vi "בדיקת זמן מיתוג הממסר 7.vi"(8 "error":errorcluster, 11 "Path for Log":path) -> (0 "error out":errorcluster, 1 "בטוח כן/לא":bool, 2 "בדיקת זמן מיתוג הממסר":dbl)   [LabVIEW 2015]
uses:
  <instrlib>/niDMM/nidmm.llb/niDMM Function.ctl
  <instrlib>/niDMM/nidmm.llb/niDMM Resolution in Digits.ctl
  <vilib>/DAQmx/write.llb/DAQmx Write (Digital Bool 1Line 1Point).vi
  <vilib>/DAQmx/create/channels.llb/DAQmx Create Channel (DO-Digital Output).vi
  <instrlib>/niDMM/nidmm.llb/niDMM Configure Measurement Digits.vi
  <vilib>/DAQmx/miscellaneous.llb/DAQmx Fill In Error Info.vi
panel:
  in  "התחל":bool
  # "Right-Click to\nexplain error"
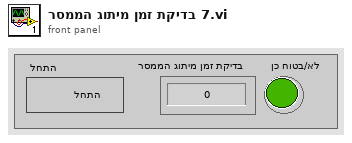
[diagram p1: front panel]
types:
  T1 = enum32{"Invalid", "Standard", "Closed", "Hidden", "Minimized", "Maximized"}
  T2 = typedef "niDMM Function.ctl" = enum16{"DC Volts", "AC Volts", "DC Current", "AC Current", "2-wire Resistance", "4-wire Resistance", "Diode", "Frequency", "Period", "AC Volts DC Coupled", "Capacitance", "Inductance", "Temperature"}
  T3 = typedef "niDMM Resolution in Digits.ctl" = dbl
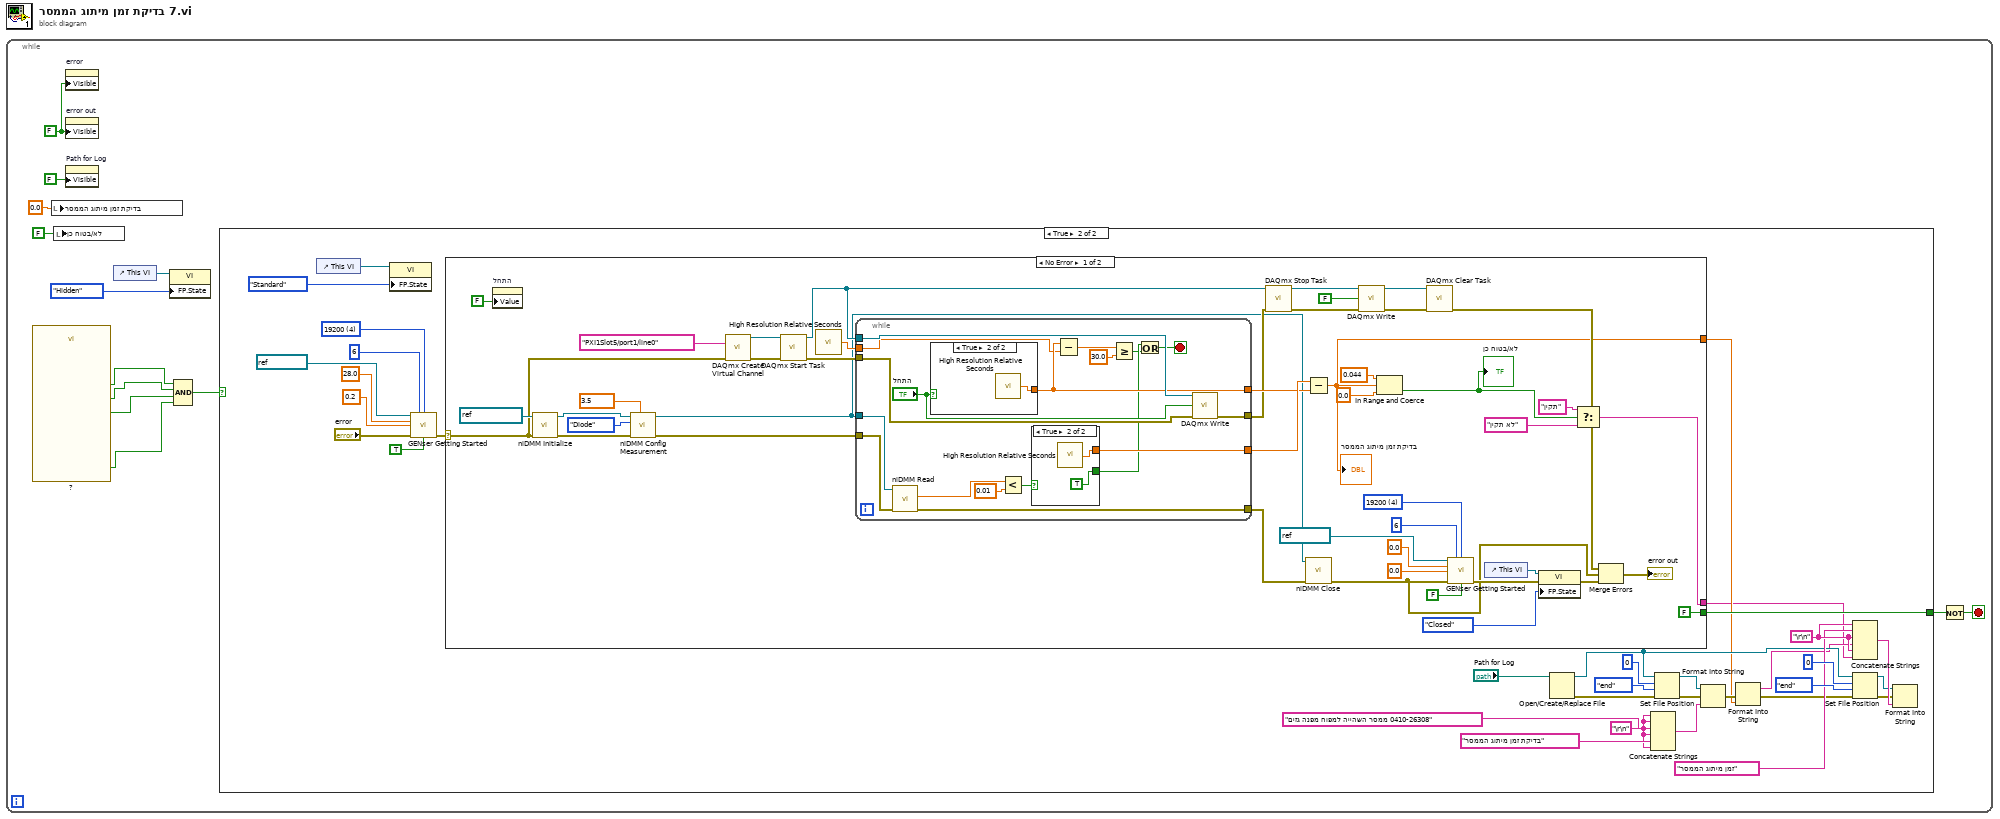
[diagram p0: block diagram]
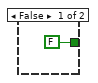
[diagram p2: hidden frame]
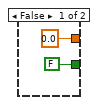
[diagram p3: hidden frame]
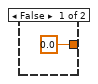
[diagram p4: hidden frame]
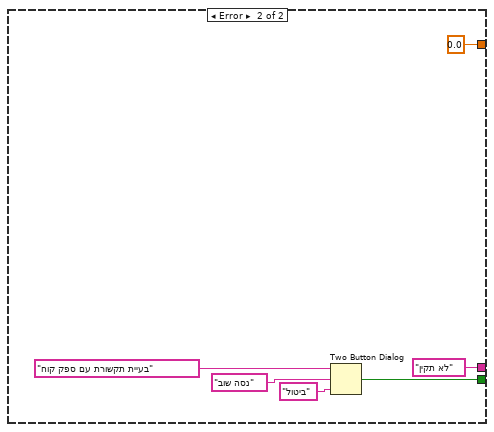
[diagram p5: hidden frame]
diagram:
  n1 = while {
    stop <- w11 stop-if-true
    w12 = FALSE ("Visible")
    n2 = call "?"() -> ("הדקי הרב מודד"=w1:bool, "(מגע שלילי (מעטפת"=w2:bool, "C מגע חיובי"=w3:bool, "OK"=w4:bool)  [unwired: 15 in, 1 out]
    n3 = local write "בדיקת זמן מיתוג הממסר"(0.0 ("בדיקת זמן מיתוג הממסר")) -> ()
    n4 = local write "בטוח כן/לא"(FALSE ("בטוח כן/לא")) -> ()
    n5 = property on="error" class="Clust (strict)"("Visible"=w12) -> ()  [unwired: 2 in, 2 out]
    n6 = property on="error out" class="Clust (strict)"("Visible"=w12) -> ()  [unwired: 2 in, 2 out]
    n7 = property on="Path for Log" class="Path"("Visible"=FALSE) -> ()  [unwired: 2 in, 2 out]
    n8 = control-ref of="This VI"() -> (w10:refnum<vi>)
    n9 = property class="VI"(reference=w10, "FP.State"=T1."Hidden" ("Front Panel Window:State")) -> ()  [unwired: 1 in, 2 out]
    n10 = Compound Arithmetic op=AND(w4, w3, w2, w1) -> (w8:bool)
    n11 = case shown="True" w8 {
      tunnel: [FALSE ("T button?") w41] -> w13
      frame False {
      }
      frame True {
        w25 = "\r\n"
        w32 = "\r\n"
        w44 = u16 4 items=["1200", "2400", "4800", "9600", "19200"] ("BAUD")
        n12 = control-ref of="This VI"() -> (w40:refnum<vi>)
        n13 = property class="VI"(reference=w40, "FP.State"=T1."Standard" ("Front Panel Window:State")) -> ()  [unwired: 1 in, 2 out]
        n14 = call "GENser Getting Started.vi"("VISA"=refnum<visa-resource-name> "COM6", "GEN Addr"=i16 6, "BAUD"=w44, "Voltage Limit"=28.0, "Current Limit"=0.2, "error"="error", "Output On (T)"=TRUE) -> ("error out"=w46:errorcluster)  [unwired: 5 in, 3 out]
        n15 = case shown="No Error" w46 {
          selector: w46 -> [w50 _]
          tunnel: [FALSE ("T button?") w120] -> w41
          tunnel: [w68 0.0] -> w17
          tunnel: [w64 "לא תקין"] -> w16
          frame No Error {
            w56 = T3 3.5 items=["3 1/2"=3.5, "4 1/2"=4.5, "5 1/2"=5.5, "6 1/2"=6.5, "7 1/2"=7.5] ("Resolution in Digits")
            w87 = u16 4 items=["1200", "2400", "4800", "9600", "19200"] ("BAUD")
            n16 = property on="התחל" class="Bool (strict)"("Value"=FALSE ("data")) -> ()  [unwired: 2 in, 2 out]
            n17 = call <instrlib>:"niDMM Initialize.vi"("error in (no error)"=w50, "Instrument Descriptor"=refnum<k15> "PXI1Slot9") -> ("error out"=w54:errorcluster, "instrument handle out"=w55:refnum<k15>)  [unwired: 8 in]
            n18 = call-poly <instrlib>:"niDMM Config Measurement.vi"("Resolution in Digits"=w56, "error in (no error)"=w54, "Function"=niDMM_Function."Diode", "instrument handle"=w55) -> ("error out"=w53:errorcluster, "instrument handle out"=w51:refnum<k15>)  [unwired: 6 in]
            n19 = call-poly <vilib>:"DAQmx Create Virtual Channel.vi"("lines"=tag "PXI1Slot5/port1/line0", "error in"=w50) -> ("task out"=w61:refnum<k21>, "error out"=w62:errorcluster)  [unwired: 12 in]
            n20 = call <vilib>:"DAQmx Start Task.vi"("task/channels in"=w61, "error in"=w62) -> ("task out"=w52:refnum<k21>, "error out"=w59:errorcluster)  [unwired: 12 in]
            n21 = call <vilib>:"High Resolution Relative Seconds.vi"() -> ("relative seconds"=w58:dbl)
            n22 = while {
              tunnel: [w103] -> w76
              tunnel: [w111] -> w77
              tunnel: [w110] -> w75
              tunnel: [w105] -> w74
              tunnel: w52 -> [w109]
              tunnel: w59 -> [w108]
              tunnel: w58 -> [w102]
              tunnel: w53 -> [w95]
              tunnel: w51 -> [w94]
              stop <- w99 stop-if-true
              n23 = call <instrlib>:"niDMM Read.vi"("error in (no error)"=w95, "instrument handle"=w94) -> ("error out"=w105:errorcluster, "Measurement"=w107:dbl)  [unwired: 7 in, 1 out]
              n24 = case shown="True" "התחל" {
                tunnel: [0.0 ("relative seconds") w117] -> w103
                frame False {
                }
                frame True {
                  n25 = call <vilib>:"High Resolution Relative Seconds.vi"() -> ("relative seconds"=w117:dbl)
                }
              }
              n26 = Less?(x=w107, y=0.01) -> (x < y?=w96:bool)
              n27 = case shown="True" w96 {
                tunnel: [0.0 ("relative seconds") w115] -> w111
                tunnel: [FALSE TRUE] -> w98
                frame False {
                }
                frame True {
                  n28 = call <vilib>:"High Resolution Relative Seconds.vi"() -> ("relative seconds"=w115:dbl)
                }
              }
              n29 = Subtract(x=w103, y=w102) -> (x-y=w101:dbl)
              n30 = Greater Or Equal?(x=w101, y=30.0) -> (x >= y?=w97:bool)
              n31 = Or(x=w98, y=w97) -> (x .or. y?=w99:bool)
              n32 = call-poly <vilib>:"DAQmx Write.vi"("task/channels in"=w109, "data"="התחל", "error in"=w108) -> ("error out"=w110:errorcluster)  [unwired: 10 in, 2 out]
            }
            n33 = call <vilib>:"DAQmx Stop Task.vi"("task/channels in"=w52, "error in"=w75) -> ("task out"=w82:refnum<k21>, "error out"=w81:errorcluster)  [unwired: 12 in]
            n34 = Subtract(x=w77, y=w76) -> (x-y=w68:dbl)
            "בדיקת זמן מיתוג הממסר" <- w68
            n35 = call <instrlib>:"niDMM Close.vi"("error in (no error)"=w74, "instrument handle"=w51) -> ("error out"=w49:errorcluster)  [unwired: 9 in]
            n36 = call-poly <vilib>:"DAQmx Write.vi"("task/channels in"=w82, "data"=FALSE, "error in"=w81) -> ("task out"=w79:refnum<k21>, "error out"=w80:errorcluster)  [unwired: 10 in, 1 out]
            n37 = In Range and Coerce(upper limit=0.044, x=w68, lower limit=0.0) -> (In Range?=w65:bool)  [unwired: 1 out]
            "בטוח כן/לא" <- w65
            n38 = call <vilib>:"DAQmx Clear Task.vi"("task in"=w79, "error in"=w80) -> ("error out"=w72:errorcluster)  [unwired: 13 in]
            n39 = call "GENser Getting Started.vi"("VISA"=refnum<visa-resource-name> "COM6", "GEN Addr"=i16 6, "BAUD"=w87, "Voltage Limit"=0.0, "Current Limit"=0.0, "error"=w49, "Output On (T)"=FALSE) -> ("error out"=w86:errorcluster)  [unwired: 5 in, 3 out]
            n40 = control-ref of="This VI"() -> (w85:refnum<vi>)
            n41 = property class="VI"(reference=w85, error in=w86, "FP.State"=T1."Closed" ("Front Panel Window:State")) -> (error out=w71:errorcluster)  [unwired: 1 out]
            n42 = Select(t="תקין", s=w65, f="לא תקין") -> (s? t:f=w64:string)
            n43 = Merge Errors(w72, w49, w71) -> (→"error out":errorcluster)
          }
          frame Error {
            n44 = Two Button Dialog(message="בעיית תקשורת עם ספק קוח", 1:"ביטול" ("F button name (\"Cancel\")"), 2:"נסה שוב" ("T button name (\"OK\")")) -> (T button?=w120:bool)
          }
        }
        n45 = Open/Create/Replace File(file path (use dialog)="Path for Log") -> (refnum out=w21:refnum<file>, error out=w22:errorcluster)  [unwired: 5 in, 1 out]
        n46 = Concatenate Strings(w32, w32, "ממסר השהייה למפוח מפנה גזים 0410-26308", w32, "בדיקת זמן מיתוג הממסר", w32) -> (w35:string)
        n47 = Set File Position(offset (in bytes) (0)=i64 0, refnum=w21, from (0:start)=enum16{"start", "end", "current"}."end", error in=w22) -> (refnum out=w33:refnum<file>, error out=w31:errorcluster)
        n48 = Format Into String(initial string=w33, error in=w31, w35) -> (error out=w20:errorcluster)  [unwired: 1 in, 1 out]
        n49 = Format Into String(error in=w20, w17) -> (resulting string=w18:string, error out=w19:errorcluster)  [unwired: 2 in]
        n50 = Concatenate Strings(w25, "זמן מיתוג הממסר", w25, w18, w25, w16) -> (w30:string)
        n51 = Set File Position(offset (in bytes) (0)=i64 0, refnum=w21, from (0:start)=enum16{"start", "end", "current"}."end", error in=w19) -> (refnum out=w28:refnum<file>, error out=w29:errorcluster)
        n52 = Format Into String(initial string=w28, error in=w29, w30) -> ()  [unwired: 1 in, 2 out]
      }
    }
    n53 = Not(x=w13) -> (.not. x?=w11:bool)
  }
